vi "S7Com_TPKT_WRT(SubVI).vi"(4 "error in":errorcluster, 5 "timeout ms":i32, 6 "TPDU_In":T1 format="X%02x", 7 "connection ID in":refnum<k5>) -> (0 "error out":errorcluster, 3 "connection ID out":refnum<k5>)   [LabVIEW 2018]
doc: "Encapsulates Transport Data Unit (TDU) into a Transport Data Packet (TPKT) and writes it."
uses:
  S7Com_HexByteArray.ctl
  S7Com_HexByte.ctl
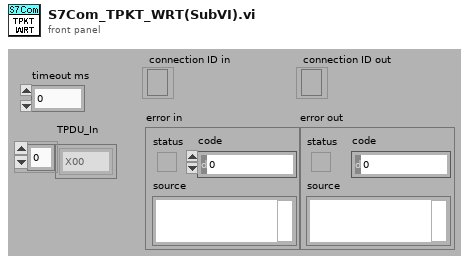
[diagram p1: front panel]
types:
  T1 = typedef "S7Com_HexByteArray.ctl" = T2[]
  T2 = typedef "S7Com_HexByte.ctl" = u8
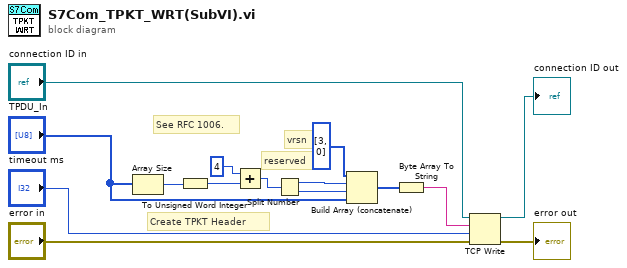
[diagram p0: block diagram]
diagram:
  # "Create TPKT Header"
  # "See RFC 1006."
  # "reserved"
  # "vrsn"
  n1 = Array Size(array="TPDU_In") -> (size(s)=w8:i32)
  n2 = To Unsigned Word Integer(number=w8) -> (unsigned 16bit integer=w9:u16)
  n3 = Add(x=u16 4, y=w9) -> (x+y=w7:u16)
  n4 = Split Number(x=w7) -> (hi(x)=w4:u8, lo(x)=w5:u8)
  n5 = Build Array (concatenate)(u8[] [3, 0], w4, w5, "TPDU_In") -> (w1:T1)
  n6 = Byte Array To String(unsigned byte array=w1) -> (string=w13:string)
  n7 = TCP Write(connection ID="connection ID in", data in=w13, error in (no error)="error in", 9:"timeout ms") -> (connection ID out=→"connection ID out":refnum<k5>, error out=→"error out":errorcluster)  [unwired: 1 out]
